vi "NIIE_Fill.vi"(6 "Color":u32(colorbox), 8 "Error":errorcluster, 9 "Point":T1={"Horizontal"=16, "Vertical"=17}, 10 "Ref Color":u32(colorbox), 11 "Data":T2={"Class"={"Ants"=refnum, "Layer"=refnum, "Templates"=refnum, "Icon"=refnum, "Glyph"=refnum, "Settings"=refnum, "Tools"=refnum}, "Ref"={"Add Layer"=refnum, "Remove Layer"=refnum, "Line Text"=[], "Body Text Spec"=refnum, "DNL_Font"=refnum, "glyph path str"=refnum, "templates path str"=refnum, "Arrow Up"=refnum, "Arrow Down"=refnum, "IE VI Ref"=refnum, "Glyphs tree"=refnum, "Templates tree"=refnum, "Layer Icon Text"=refnum, "Layer Template"=refnum, "Clipboard"=refnum, "BW icon in"=refnum, "Color icon in"=refnum, "Layer Clust"=refnum, "Body Text"=refnum, "DNL_Framework Templates"=refnum, "Search Templates"=refnum, "TextMarker"=refnum, "Tab Control"=refnum, "Search Glyphs"=refnum, "Line Color"=refnum, "DNL_Glyphs []"=refnum, "Fill Color"=refnum, "Tools"=refnum, "Glyphs tree"=refnum, "Icon"=refnum, "Preview"=refnum, "Ants"=refnum, "Terminals"=refnum, "menu reference"=refnum, "LayerNames"=[], "GlyphLoadAnimation"=refnum, "TemplateLoadAnimation"=refnum, "refreshGlyphs"=refnum, "refreshTemplates"=refnum}, "Support"={"AntsRect"={"left"=0, "top"=0, "right"=0, "bottom"=0}, "Mouse Move Coords"={"Horizontal"=0, "Vertical"=0}, "Mouse Down Coords"={"Horizontal"=0, "Vertical"=0}, "Temp Coord"={"Horizontal"=0, "Vertical"=0}, "Action"=enum."Default", "Edge Color"=4914962, "Fill Color"=16860, "Mouse Down?"=FALSE, "Draft Mode?"=FALSE, "Temp Icon"=bytes[3102], "CTRL Pressed"=FALSE, "Move Selection?"=FALSE, "AntsRect Orig"={"left"=0, "top"=0, "right"=0, "bottom"=0}, "Text"="", "TM Set?"=FALSE, "Mouse inside icon?"=FALSE, "Tool (old value)"=0, "Pencil Move Color"=0, "Swap Colors?"=FALSE, "Shift pressed?"=FALSE}}) -> (0 "Error Out":errorcluster, 3 "Data Out":T2={"Class"={"Ants"=refnum, "Layer"=refnum, "Templates"=refnum, "Icon"=refnum, "Glyph"=refnum, "Settings"=refnum, "Tools"=refnum}, "Ref"={"Add Layer"=refnum, "Remove Layer"=refnum, "Line Text"=[], "Body Text Spec"=refnum, "DNL_Font"=refnum, "glyph path str"=refnum, "templates path str"=refnum, "Arrow Up"=refnum, "Arrow Down"=refnum, "IE VI Ref"=refnum, "Glyphs tree"=refnum, "Templates tree"=refnum, "Layer Icon Text"=refnum, "Layer Template"=refnum, "Clipboard"=refnum, "BW icon in"=refnum, "Color icon in"=refnum, "Layer Clust"=refnum, "Body Text"=refnum, "DNL_Framework Templates"=refnum, "Search Templates"=refnum, "TextMarker"=refnum, "Tab Control"=refnum, "Search Glyphs"=refnum, "Line Color"=refnum, "DNL_Glyphs []"=refnum, "Fill Color"=refnum, "Tools"=refnum, "Glyphs tree"=refnum, "Icon"=refnum, "Preview"=refnum, "Ants"=refnum, "Terminals"=refnum, "menu reference"=refnum, "LayerNames"=[], "GlyphLoadAnimation"=refnum, "TemplateLoadAnimation"=refnum, "refreshGlyphs"=refnum, "refreshTemplates"=refnum}, "Support"={"AntsRect"={"left"=0, "top"=0, "right"=0, "bottom"=0}, "Mouse Move Coords"={"Horizontal"=0, "Vertical"=0}, "Mouse Down Coords"={"Horizontal"=0, "Vertical"=0}, "Temp Coord"={"Horizontal"=0, "Vertical"=0}, "Action"=enum."Default", "Edge Color"=4914962, "Fill Color"=16860, "Mouse Down?"=FALSE, "Draft Mode?"=FALSE, "Temp Icon"=bytes[3102], "CTRL Pressed"=FALSE, "Move Selection?"=FALSE, "AntsRect Orig"={"left"=0, "top"=0, "right"=0, "bottom"=0}, "Text"="", "TM Set?"=FALSE, "Mouse inside icon?"=FALSE, "Tool (old value)"=0, "Pencil Move Color"=0, "Swap Colors?"=FALSE, "Shift pressed?"=FALSE}})   [LabVIEW 2021]
uses:
  Controls/IE Data.ctl
  Class/Ants/Ants.lvclass
  Class/FakedArray/FakedArray.lvclass
  vi.lib/LabVIEW Icon API/lv_icon/Classes/Icon/Icon.lvclass
  Class/Icon Library/Glyph.lvclass
  Class/Settings/Settings.lvclass
  Class/Tools/Tools Paint.lvclass
  Controls/IE Classes.ctl
  Controls/References Cluster.ctl
  Controls/SupportClass.ctl
  <vilib>/Utility/miscctls.llb/LVPoint32TypeDef.ctl
  Controls/ENUM_SupportClass_Action.ctl
  vi.lib/LabVIEW Icon API/lv_icon/Controls/IEColor.ctl
  vi.lib/LabVIEW Icon API/lv_icon/Controls/LayerType.ctl
  vi.lib/LabVIEW Icon API/lv_icon/Classes/Layer/Layer.lvclass
  vi.lib/LabVIEW Icon API/lv_icon/Classes/Icon Framework/Icon Framework.lvclass
  C:/Users/Mark.Balla/Projects/MB Tools/ICON Editor LV/labview-icon-editor-main LV2021 2024-10-24/vi.lib/LabVIEW Icon API/lv_icon/classes/Layer/Layer.lvclass
  vi.lib/LabVIEW Icon API/lv_icon/lv_icon.lvlib
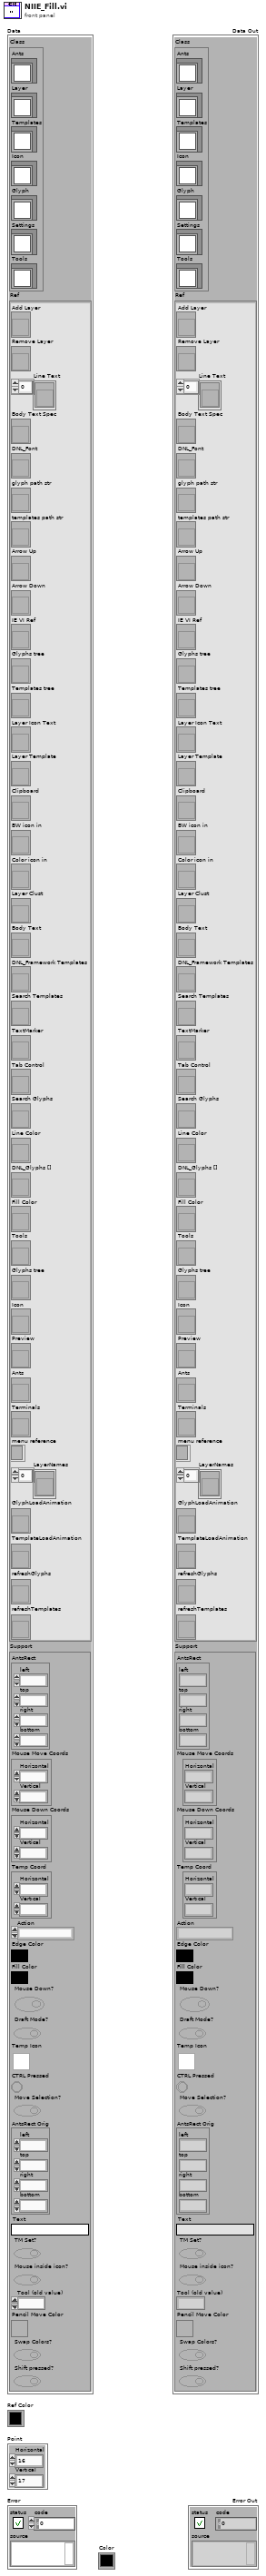
[diagram p1: front panel]
types:
  T1 = typedef "LVPoint32TypeDef.ctl" = cluster{"Horizontal":i32, "Vertical":i32}
  T2 = typedef "IE Data.ctl" = cluster{"Class":T3, "Ref":T4, "Support":T5}
  T3 = typedef "IE Classes.ctl" = cluster{"Ants":refnum<class "Ants.lvclass">, "Layer":refnum<class "FakedArray.lvclass">, "Templates":refnum<class "FakedArray.lvclass">, "Icon":refnum<class "Icon.lvclass">, "Glyph":refnum<class "Glyph.lvclass">, "Settings":refnum<class "Settings.lvclass">, "Tools":refnum<class "Tools Paint.lvclass">}
  T4 = typedef "References Cluster.ctl" = cluster{"Add Layer":refnum<vi>, "Remove Layer":refnum<vi>, "Line Text":refnum<vi>[], "Body Text Spec":refnum<vi>, "DNL_Font":refnum<vi>, "glyph path str":refnum<vi>, "templates path str":refnum<vi>, "Arrow Up":refnum<vi>, "Arrow Down":refnum<vi>, "IE VI Ref":refnum<vi>, "Glyphs tree":refnum<vi>, "Templates tree":refnum<vi>, "Layer Icon Text":refnum<vi>, "Layer Template":refnum<vi>, "Clipboard":refnum<vi>, "BW icon in":refnum<vi>, "Color icon in":refnum<vi>, "Layer Clust":refnum<vi>, "Body Text":refnum<vi>, "DNL_Framework Templates":refnum<vi>, "Search Templates":refnum<vi>, "TextMarker":refnum<vi>, "Tab Control":refnum<vi>, "Search Glyphs":refnum<vi>, "Line Color":refnum<vi>, "DNL_Glyphs []":refnum<vi>, "Fill Color":refnum<vi>, "Tools":refnum<vi>, "Glyphs tree":refnum<vi>, "Icon":refnum<vi>, "Preview":refnum<vi>, "Ants":refnum<vi>, "Terminals":refnum<vi>, "menu reference":refnum<k9>, "LayerNames":refnum<vi>[], "GlyphLoadAnimation":refnum<vi>, "TemplateLoadAnimation":refnum<vi>, "refreshGlyphs":refnum<vi>, "refreshTemplates":refnum<vi>}
  T5 = typedef "SupportClass.ctl" = cluster{"AntsRect":cluster{"left":i16, "top":i16, "right":i16, "bottom":i16}, "Mouse Move Coords":T1, "Mouse Down Coords":T1, "Temp Coord":T1, "Action":T6, "Edge Color":T7, "Fill Color":T7, "Mouse Down?":bool, "Draft Mode?":bool, "Temp Icon":picture, "CTRL Pressed":bool, "Move Selection?":bool, "AntsRect Orig":cluster{"left":i16, "top":i16, "right":i16, "bottom":i16}, "Text":string, "TM Set?":bool, "Mouse inside icon?":bool, "Tool (old value)":u32, "Pencil Move Color":u32, "Swap Colors?":bool, "Shift pressed?":bool}
  T6 = typedef "ENUM_SupportClass_Action.ctl" = enum16{"Default", "Move Selection", "Glyph Library", "Tool"}
  T7 = typedef "IEColor.ctl" = u32
  T8 = typedef "LayerType.ctl" = enum16{"Graphic", "Text", "Tool", "Graphic Drop"}
  T9 = typedef "Cluster_INI Data.ctl" = cluster{"Show Layer Tab?":bool, "Show Terminals?":bool, "Text":cluster{"Font":T10, "Alignment":T11, "Size":T12}, "3rd party Templates":cluster{"Store 3rd party Templates?":bool, "Folder Name":string}, "Merge user layers on commit":bool, "Body Text":T13, "Fill Color":T7, "Edge Color":T7, "Tab":u16, "Tool":T14, "Disable Layers?":bool}
  T10 = typedef "Font.ctl" = string
  T11 = typedef "Alignment.ctl" = u16
  T12 = typedef "Num_Font Size.ctl" = u8
  T13 = typedef "Cluster_BodyText.ctl" = cluster{"Line 1 text":string, "Line 2 text":string, "Line 3 text":string, "Line 4 text":string, "Line 1 color":u32, "Line 2 color":u32, "Line 3 color":u32, "Line 4 color":u32, "Body Text Spec":cluster{"Font":T10, "Alignment":T11, "Size":u8}, "Center text vertically":bool, "Capitalize Text":bool}
  T14 = typedef "Cluster_Button Draw Tools.ctl" = enum32{"Pencil", "Line", "Dropper", "Fill", "Rectangle", "Filled Rectangle", "Ellipse", "Filled Ellipse", "Eraser", "Text", "Select", "Move"}
  T15 = typedef "Cluster_Layer Data.ctl" = cluster{"LayerIcon":picture, "LayerName":string, "Opacity":u8, "Visibility?":bool}
  T16 = typedef "LVPositionTypeDef.ctl" = cluster{"Left":i32, "Top":i32}
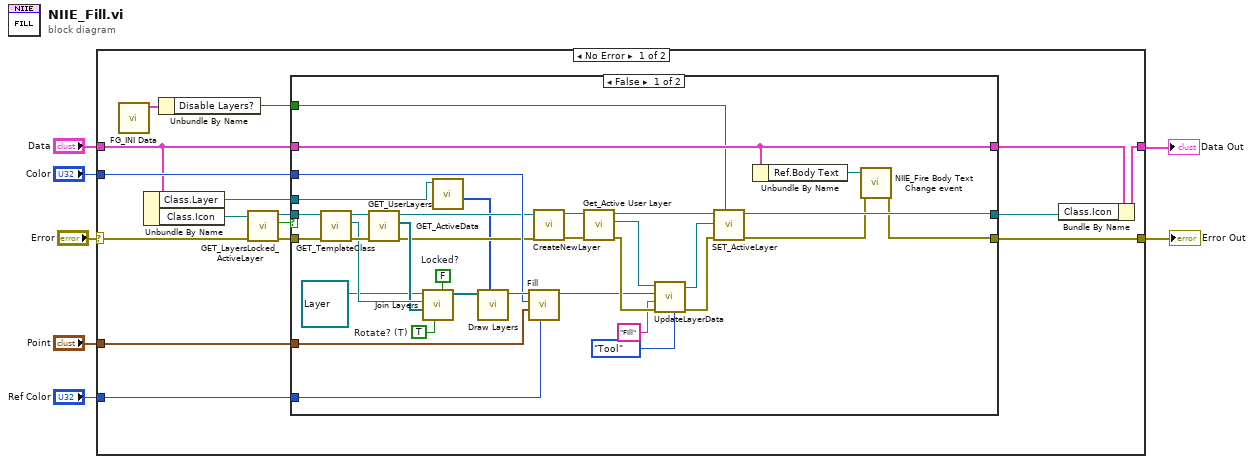
[diagram p0: block diagram]
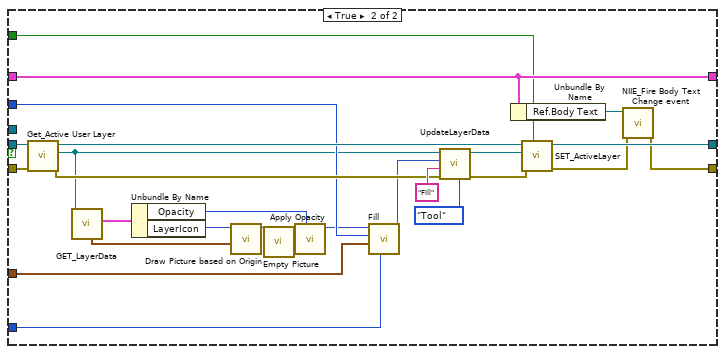
[diagram p2: hidden frame]
diagram:
  n1 = case shown="No Error" "Error" {
    selector: "Error" -> [w17 w85]
    tunnel: [w13 w85] -> w6
    tunnel: "Point" -> [w23 _]
    tunnel: "Color" -> [w19 _]
    tunnel: "Ref Color" -> [w18 _]
    tunnel: "Data" -> [w15 w84]
    tunnel: [w12 w84] -> w2
    frame No Error {
      n2 = call "FG_INI Data.vi"() -> ("INI Data Out"=w9:T9)  [unwired: 1 in, 10 out]
      n3 = Unbundle By Name(w15) -> ("Class.Layer"=w10:refnum<class "FakedArray.lvclass">, "Class.Icon"=w16:refnum<class "Icon.lvclass">)
      n4 = Unbundle By Name(w9) -> ("Disable Layers?"=w8:bool)
      n5 = call-dynamic "GET_LayersLocked_ActiveLayer.vi"("error in (no error)"=w17, "Icon.lvclass in"=w16) -> ("error out"=w21:errorcluster, "Layers Locked?"=w20:bool, "Icon.lvclass out"=w22:refnum<class "Icon.lvclass">)  [unwired: 7 out]
      n6 = case shown="False" w20 {
        tunnel: w23 -> [w48 w74]
        tunnel: [w34 w81] -> w11
        tunnel: w22 -> [w56 w83]
        tunnel: w21 -> [w57 w82]
        tunnel: w19 -> [w49 w75]
        tunnel: w18 -> [w50 w73]
        tunnel: [w31 w60] -> w13
        tunnel: w15 -> [w30 w62]
        tunnel: [w30 w62] -> w14
        tunnel: w10 -> [w27 _]
        tunnel: w8 -> [w28 w58]
        frame False {
          w24 = FALSE  # Locked?
          w25 = TRUE  # Rotate? (T)
          n7 = call-dynamic "GET_TemplateClass.vi"("error in (no error)"=w57, "Icon.lvclass in"=w56) -> ("error out"=w55:errorcluster, "Icon Framework.lvclass"=w53:refnum<class "Icon Framework.lvclass">, "Icon.lvclass out"=w54:refnum<class "Icon.lvclass">)  [unwired: 7 out]
          n8 = call-dynamic "GET_UserLayers.vi"("error in (no error)"=w55, "Icon.lvclass in"=w54) -> ("error out"=w36:errorcluster, "All Layers"=w47:refnum<class "Layer.lvclass">[], "Icon.lvclass out"=w37:refnum<class "Icon.lvclass">)  [unwired: 7 out]
          n9 = call "Join Layers.vi"("Locked?"=w24, "Rotate? (T)"=w25, "User Layers"=w47, "Template"=w53, "Icon Text"=refnum<class "Layer.lvclass"> refnum) -> ("Layer Out"=w52:refnum<class "Layer.lvclass">[])  [unwired: 1 in, 5 out]
          n10 = call-dynamic "GET_ActiveData.vi"("FakedArray"=w27) -> ("Active Data [] Out"=w26:i32[])  [unwired: 5 in, 5 out]
          n11 = call "Draw Layers.vi"("Active User Layer Data []"=w26, "Layers"=w52) -> ("Picture"=w51:picture)  [unwired: 3 in, 6 out]
          n12 = call "Fill.vi"("Ref Color"=w50, "Pic Mouse Down"=w48, "New Color"=w49, "Pic"=w51) -> ("Pic Out"=w35:picture)  [unwired: 3 in, 4 out]
          n13 = call "CreateNewLayer.vi"("error in"=w36, "Icon.lvclass"=w37) -> ("error out"=w45:errorcluster, "Icon.lvclass out"=w46:refnum<class "Icon.lvclass">)  [unwired: 3 in, 5 out]
          n14 = call-dynamic "Get_Active User Layer.vi"("error in (no error)"=w45, "Icon in"=w46) -> ("error out"=w40:errorcluster, "Layer.lvclass"=w44:refnum<class "Layer.lvclass">, "Icon out"=w43:refnum<class "Icon.lvclass">)  [unwired: 7 out]
          n15 = call "UpdateLayerData.vi"("Type"=LayerType."Tool", "error in"=w40, "LayerName"="Fill" ("FileName"), "new picture"=w35, "Active Layer"=w44) -> ("error out"=w41:errorcluster, "Layer.lvclass out"=w42:refnum<class "Layer.lvclass">)  [unwired: 3 in, 2 out]
          n16 = call-dynamic "SET_ActiveLayer.vi"("Combine User Layers?"=w28, "Error"=w41, "Layer.lvclass"=w42, "Icon.lvclass"=w43) -> ("Error Out"=w32:errorcluster, "Icon.lvclass Out"=w34:refnum<class "Icon.lvclass">)  [unwired: 6 out]
          n17 = Unbundle By Name(w30) -> ("Ref.Body Text"=w29:refnum<vi>)
          n18 = call "NIIE_Fire Body Text Change event.vi"("error in"=w32, "Ref.Body Text"=w29) -> ("error out"=w31:errorcluster)  [unwired: 2 in, 7 out]
        }
        frame True {
          n19 = call-dynamic "Get_Active User Layer.vi"("error in (no error)"=w82, "Icon in"=w83) -> ("error out"=w77:errorcluster, "Layer.lvclass"=w68:refnum<class "Layer.lvclass">, "Icon out"=w80:refnum<class "Icon.lvclass">)  [unwired: 7 out]
          n20 = call-dynamic "GET_LayerData.vi"("Layer.lvclass in"=w68) -> ("Data"=w67:T15, "Origin"=w65:T16)  [unwired: 1 in, 8 out]
          n21 = Unbundle By Name(w67) -> ("Opacity"=w64:u8, "LayerIcon"=w66:picture)
          n22 = call "Draw Picture based on Origin.vi"("Origin"=w65, "LayerIcon in"=w66) -> ("LayerIcon out"=w69:picture)  [unwired: 1 in, 8 out]
          n23 = call "Empty Picture"() -> ("empty picture"=w70:picture)
          n24 = call "Apply Opacity.vi"("% (100)"=w64, "Bottom"=w70, "Top"=w69) -> ("new picture"=w63:picture)  [unwired: 8 out]
          n25 = call "Fill.vi"("Ref Color"=w73, "Pic Mouse Down"=w74, "New Color"=w75, "Pic"=w63) -> ("Pic Out"=w72:picture)  [unwired: 3 in, 4 out]
          n26 = call "UpdateLayerData.vi"("Type"=LayerType."Tool", "error in"=w77, "LayerName"="Fill" ("Fill"), "new picture"=w72, "Active Layer"=w68) -> ("error out"=w76:errorcluster, "Layer.lvclass out"=w71:refnum<class "Layer.lvclass">)  [unwired: 3 in, 2 out]
          n27 = Unbundle By Name(w62) -> ("Ref.Body Text"=w59:refnum<vi>)
          n28 = call-dynamic "SET_ActiveLayer.vi"("Combine User Layers?"=w58, "Error"=w76, "Layer.lvclass"=w71, "Icon.lvclass"=w80) -> ("Error Out"=w61:errorcluster, "Icon.lvclass Out"=w81:refnum<class "Icon.lvclass">)  [unwired: 6 out]
          n29 = call "NIIE_Fire Body Text Change event.vi"("error in"=w61, "Ref.Body Text"=w59) -> ("error out"=w60:errorcluster)  [unwired: 2 in, 7 out]
        }
      }
      n30 = Bundle By Name(cluster=w14, "Class.Icon"=w11) -> (w12:T2)
    }
    frame Error {
    }
  }
  "Error Out" <- w6
  "Data Out" <- w2
